vi "Calc IoU.vi"(10 "Box_2":T1={"conf"=0.986422, "x_center"=631.1553, "y_center"=551.02734, "width"=680.6134, "height"=681.4035, "x1"=290.84857, "y1"=210.32559, "x2"=971.462, "y2"=891.7291}, 11 "Box_1":T1={"conf"=0.987858, "x_center"=630.68286, "y_center"=551.3997, "width"=681.5454, "height"=679.5936, "x1"=289.91016, "y1"=211.6029, "x2"=971.45557, "y2"=891.19653}) -> (3 "IoU":sgl)   [LabVIEW 2017, in "postprocess_YOLOv8.lvlib"]
uses:
  postprocess_YOLOv8.lvlib
  Box.ctl
panel:
  out "area_2":sgl
  out "area_1":sgl
  out "intersection area":sgl
  out "y_bottom":sgl
  out "x_right":sgl
  out "y_top":sgl
  out "x_left":sgl
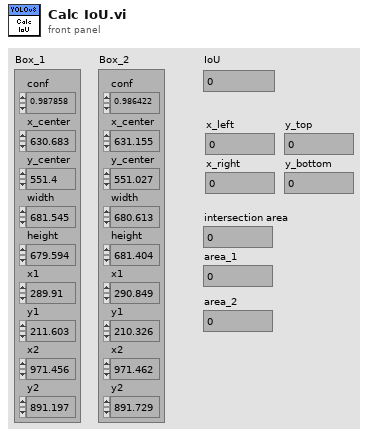
[diagram p1: front panel]
types:
  T1 = typedef "postprocess_YOLOv8.lvlib/Box.ctl" = cluster{"conf":sgl, "x_center":sgl, "y_center":sgl, "width":sgl, "height":sgl, "x1":sgl, "y1":sgl, "x2":sgl, "y2":sgl}
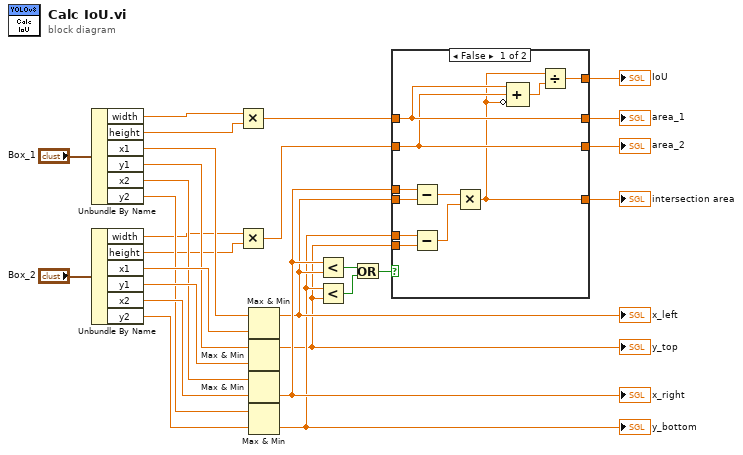
[diagram p0: block diagram]
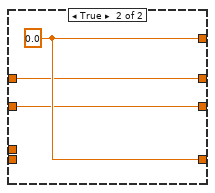
[diagram p2: hidden frame]
diagram:
  n1 = Unbundle By Name("Box_1") -> ("width"=w8:sgl, "height"=w7:sgl, "x1"=w25:sgl, "y1"=w23:sgl, "x2"=w21:sgl, "y2"=w19:sgl)
  n2 = Unbundle By Name("Box_2") -> ("width"=w6:sgl, "height"=w5:sgl, "x1"=w24:sgl, "y1"=w22:sgl, "x2"=w20:sgl, "y2"=w18:sgl)
  n3 = Multiply(x=w8, y=w7) -> (x*y=w4:sgl)
  n4 = Multiply(x=w6, y=w5) -> (x*y=w1:sgl)
  n5 = Max & Min(x=w25, y=w24) -> (max(x,y)=w12:sgl)  [unwired: 1 out]
  "x_left" <- w12
  n6 = Max & Min(x=w23, y=w22) -> (max(x,y)=w10:sgl)  [unwired: 1 out]
  "y_top" <- w10
  n7 = Max & Min(x=w21, y=w20) -> (min(x,y)=w13:sgl)  [unwired: 1 out]
  "x_right" <- w13
  n8 = Max & Min(x=w19, y=w18) -> (min(x,y)=w11:sgl)  [unwired: 1 out]
  "y_bottom" <- w11
  n9 = Less?(x=w13, y=w12) -> (x < y?=w17:bool)
  n10 = Less?(x=w11, y=w10) -> (x < y?=w16:bool)
  n11 = Or(x=w17, y=w16) -> (x .or. y?=w15:bool)
  n12 = case shown="False" w15 {
    tunnel: [w28 w41] -> w14
    tunnel: w13 -> [w38 _]
    tunnel: w12 -> [w37 _]
    tunnel: w11 -> [w36 _]
    tunnel: w10 -> [w35 _]
    tunnel: [w30 w41] -> w9
    tunnel: w4 -> [w32 w40]
    tunnel: [w32 w40] -> w3
    tunnel: w1 -> [w31 w39]
    tunnel: [w31 w39] -> w2
    frame False {
      n13 = Subtract(x=w38, y=w37) -> (x-y=w34:sgl)
      n14 = Subtract(x=w36, y=w35) -> (x-y=w33:sgl)
      n15 = Multiply(x=w34, y=w33) -> (x*y=w30:sgl)
      n16 = Compound Arithmetic op=ADD(w32, w31, invert w30) -> (w29:sgl)
      n17 = Divide(x=w30, y=w29) -> (x/y=w28:sgl)
    }
    frame True {
      w41 = sgl 0.0
    }
  }
  "IoU" <- w14
  "intersection area" <- w9
  "area_1" <- w3
  "area_2" <- w2
